vi "Test Python String to LabVIEW Data.vi"() -> ()   [LabVIEW 2020, in "jki_python_data_tools.lvlib"]
uses:
  jki_python_data_tools.lvlib
  LabVIEW Data to Python String/LabVIEW Data to Python String (Variant).vi
  Python String to LabVIEW Data/Python String to LabVIEW Data (Variant).vi
panel:
  in  "Theta (All Field Vectors)[] 2":cluster{"Theta(Field Vector)[]":dbl[]}[](array[cluster])
  out "Theta (All Field Vectors)[]":cluster{"Theta(Field Vector)[]":dbl[]}[](array[cluster])
  out "Python String  2":string
  out "x = y?":bool
  out "error out":errorcluster
  in  "All Field Vectors[] 3":T1(array[cluster])=[{"Field Vector[]"=[{"Signal Index []"=[0, 1]}, {"Signal Index []"=[2, 3]}, {"Signal Index []"=[4, 5]}, {"Signal Index []"=[6, 7]}, {"Signal Index []"=[8, 9]}, {"Signal Index []"=[10, 11]}, {"Signal Index []"=[12, 13]}, {"Signal Index []"=[14]}, {"Signal Index []"=[15]}]}, {"Field Vector[]"=[{"Signal Index []"=[16, 17]}, {"Signal Index []"=[18, 19]}, {"Signal Index []"=[20, 21]}, {"Signal Index []"=[22, 23]}, {"Signal Index []"=[24, 25]}, {"Signal Index []"=[26, 27]}, {"Signal Index []"=[28, 29]}, {"Signal Index []"=[30]}, {"Signal Index []"=[31]}]}, {"Field Vector[]"=[{"Signal Index []"=[32, 33]}, {"Signal Index []"=[34, 35]}, {"Signal Index []"=[36, 37]}, {"Signal Index []"=[38, 39]}, {"Signal Index []"=[40, 41]}, {"Signal Index []"=[42, 43]}, {"Signal Index []"=[44, 45]}, {"Signal Index []"=[46]}, {"Signal Index []"=[47]}]}]
  out "LabVIEW Data":variant
  out "Python String":string
  # "Copyright © 2003-2009 JKI. All rights reserved.\n\nAuthor: Jim Kring [jim.kring@jameskring.com]\n\nThis library is provided \"AS IS\" ,WITHOUT WARRANTIES OR \nCONDITIONS OF ANY KIND, either express or implied.\n\nJames Kring, Inc. -- http://www.jameskring.com"
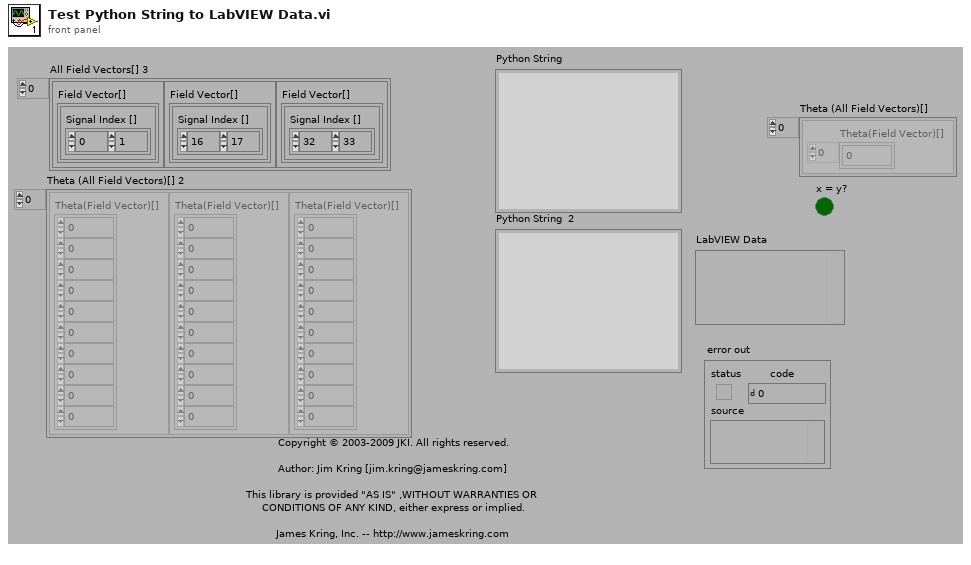
[diagram p1: front panel]
types:
  T1 = cluster{"Field Vector[]":cluster{"Signal Index []":u8[]}[]}[]
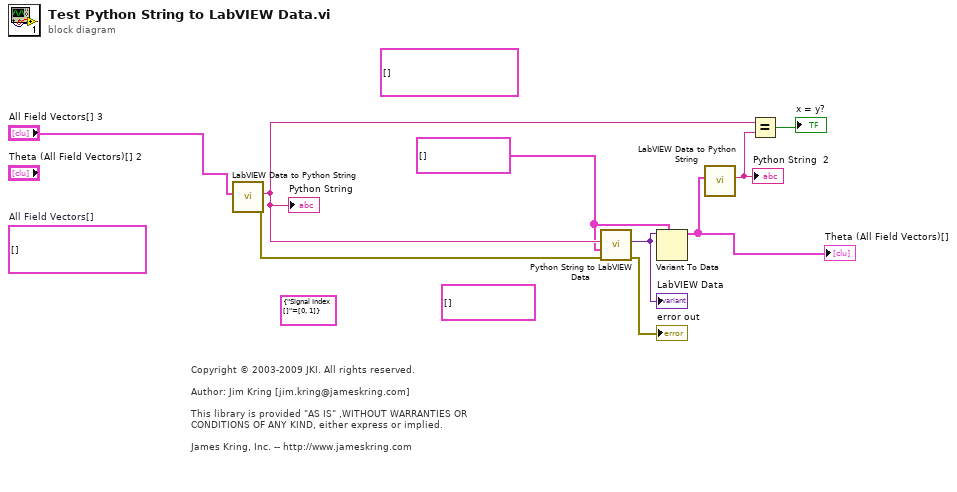
[diagram p0: block diagram]
diagram:
  (unwired) T1 [] ("All Field Vectors[] 3")
  w3 = cluster{"Theta(Field Vector)[]":dbl[]}[] [] ("Theta (All Field Vectors)[]")
  (unwired) cluster{"Signal Index []":u8[]}[] [] ("Field Vector[]")
  (unwired) cluster{"Signal Index []":u8[]} {"Signal Index []"=[0, 1]} ("Signal Pair")
  (unwired) T1 []  # All Field Vectors[]
  # "Copyright © 2003-2009 JKI. All rights reserved.\n\nAuthor: Jim Kring [jim.kring@jameskring.com]\n\nThis library is provided \"AS IS\" ,WITHOUT WARRANTIES OR \nCONDITIONS OF ANY KIND, either express or implied.\n\nJames Kring, Inc. -- http://www.jameskring.com"
  n1 = call-poly "LabVIEW Data to Python String.vi"("LabVIEW Data"="All Field Vectors[] 3") -> ("error out"=w8:errorcluster, "Python String"=w6:string)  [unwired: 9 in]
  "Python String" <- w6
  n2 = call-poly "Python String to LabVIEW Data.vi"("error in (no error)"=w8, "type"=w3, "Python String"=w6) -> ("error out"=→"error out":errorcluster, "LabVIEW Data"=w5:variant)  [unwired: 7 in]
  "LabVIEW Data" <- w5
  n3 = Variant To Data(type=w3, Variant=w5) -> (data=w2:cluster{"Theta(Field Vector)[]":dbl[]}[])  [unwired: 1 in, 1 out]
  "Theta (All Field Vectors)[]" <- w2
  n4 = call-poly "LabVIEW Data to Python String.vi"("LabVIEW Data"=w2) -> ("Python String"=w4:string)  [unwired: 9 in, 1 out]
  "Python String  2" <- w4
  n5 = Equal?(x=w6, y=w4) -> (x = y?=→"x = y?":bool)
